vi "Activate Menu.vi"(8 "error in (no error)":errorcluster, 9 "Run mode?":bool, 10 "MenuRef":refnum<k9>, 11 "2D Plotmatrix.lvclass in":refnum<class "XY Plot Matrix.lvclass">) -> (0 "error out":errorcluster, 3 "2D Plotmatrix.lvclass out":refnum<class "XY Plot Matrix.lvclass">)   [LabVIEW 2020, in "XY Plot Matrix.lvclass"]
uses:
  <vilib>/Math Plots/2D Math Plots/XY Plot Matrix/XY Plot Matrix/XY Plot Matrix.lvclass
  e:/builds/penguin/labview/branches/2020/dev/dist/vi.lib/Math Plots/2D Math Plots/2D Plot/2D Plot/2D Plot.lvclass
  <vilib>/Math Plots/2D Math Plots/2D Plot/2D Plot/2D Plot.lvclass
panel:
  in  "Run-time Menu":T1(array[cluster])=[{"menu tag"="", "items to delete"=["APP_SC_AUTOSCALE_X", "APP_SC_AUTOSCALE_Y", "APP_SC_SMOOTH_UPDATES", "APP_SC_OPTIONAL_PLANE", "APP_SC_EXPORT", "APP_SC_SHOW_DIAGRAM", "APP_SC_EXPORT_SIMPLIFIED_IMAGE"], "new menu"=[{"item names"="Autoscale X", "item tags"="USER_SC_AUTOSCALE_X", "after item"="APP_SC_AUTOSCALE_X"}, {"item names"="Autoscale Y", "item tags"="USER_SC_AUTOSCALE_Y", "after item"="USER_SC_AUTOSCALE_X"}, {"item names"="Export Simplified Image...", "item tags"="USER_SC_EXPORT_SIMPLIFIED_IMAGE", "after item"="APP_SC_VISIBLE_ITEMS"}], "root?"=TRUE}, {"menu tag"="APP_SC_VISIBLE_ITEMS", "items to delete"=["APP_SC_PLOT_LEGEND", "APP_SC_SCALE_LEGEND", "APP_SC_GRAPH_PALETTE", "APP_SC_CURSOR_LEGEND", "APP_SC_X_SCROLLBAR", "APP_SC_X_SCALE", "APP_SC_Y_SCALE", "APP_SC_UNIT_LABEL"], "new menu"=[{"item names"="Plot Legend", "item tags"="USER_SC_PLOT_LEGEND", "after item"="APP_SC_SEPERATOR"}, {"item names"="Graph Palette", "item tags"="USER_SC_GRAPH_PALETTE", "after item"="USER_SC_SCALE_LEGEND"}], "root?"=FALSE}]
  in  "Edit-time Menu":T1(array[cluster])=[{"menu tag"="", "items to delete"=["APP_SC_AUTOSCALE_X", "APP_SC_AUTOSCALE_Y", "APP_SC_SMOOTH_UPDATES", "APP_SC_OPTIONAL_PLANE", "APP_SC_EXPORT", "APP_SC_PROPERTIES", "APP_SC_EXPORT_SIMPLIFIED_IMAGE"], "new menu"=[{"item names"="Autoscale X", "item tags"="USER_SC_AUTOSCALE_X", "after item"="APP_SC_AUTOSCALE_X"}, {"item names"="Autoscale Y", "item tags"="USER_SC_AUTOSCALE_Y", "after item"="USER_SC_AUTOSCALE_X"}, {"item names"="Export Simplified Image...", "item tags"="USER_SC_EXPORT_SIMPLIFIED_IMAGE", "after item"="APP_SC_OPTIONAL_PLANE"}, {"item names"="Properties", "item tags"="USER_SC_PROPERTIES", "after item"="APP_SC_PROPERTIES"}, {"item names"="", "item tags"="", "after item"=""}, {"item names"="", "item tags"="", "after item"=""}, {"item names"="", "item tags"="", "after item"=""}, {"item names"="", "item tags"="", "after item"=""}, {"item names"="", "item tags"="", "after item"=""}, {"item names"="Autoscale X", "item tags"="USER_SC_AUTOSCALE_X", "after item"="APP_SC_AUTOSCALE_X"}], "root?"=TRUE}, {"menu tag"="APP_SC_VISIBLE_ITEMS", "items to delete"=["APP_SC_PLOT_LEGEND", "APP_SC_SCALE_LEGEND", "APP_SC_GRAPH_PALETTE", "APP_SC_CURSOR_LEGEND", "APP_SC_X_SCROLLBAR", "APP_SC_X_SCALE", "APP_SC_Y_SCALE", "APP_SC_UNIT_LABEL"], "new menu"=[{"item names"="Plot Legend", "item tags"="USER_SC_PLOT_LEGEND", "after item"="APP_SC_SEPERATOR"}, {"item names"="Graph Palette", "item tags"="USER_SC_GRAPH_PALETTE", "after item"="USER_SC_SCALE_LEGEND"}], "root?"=FALSE}, {"menu tag"="APP_SC_ADVANCED", "items to delete"=["APP_SC_SHOW_DIAGRAM"], "new menu"=[], "root?"=FALSE}]
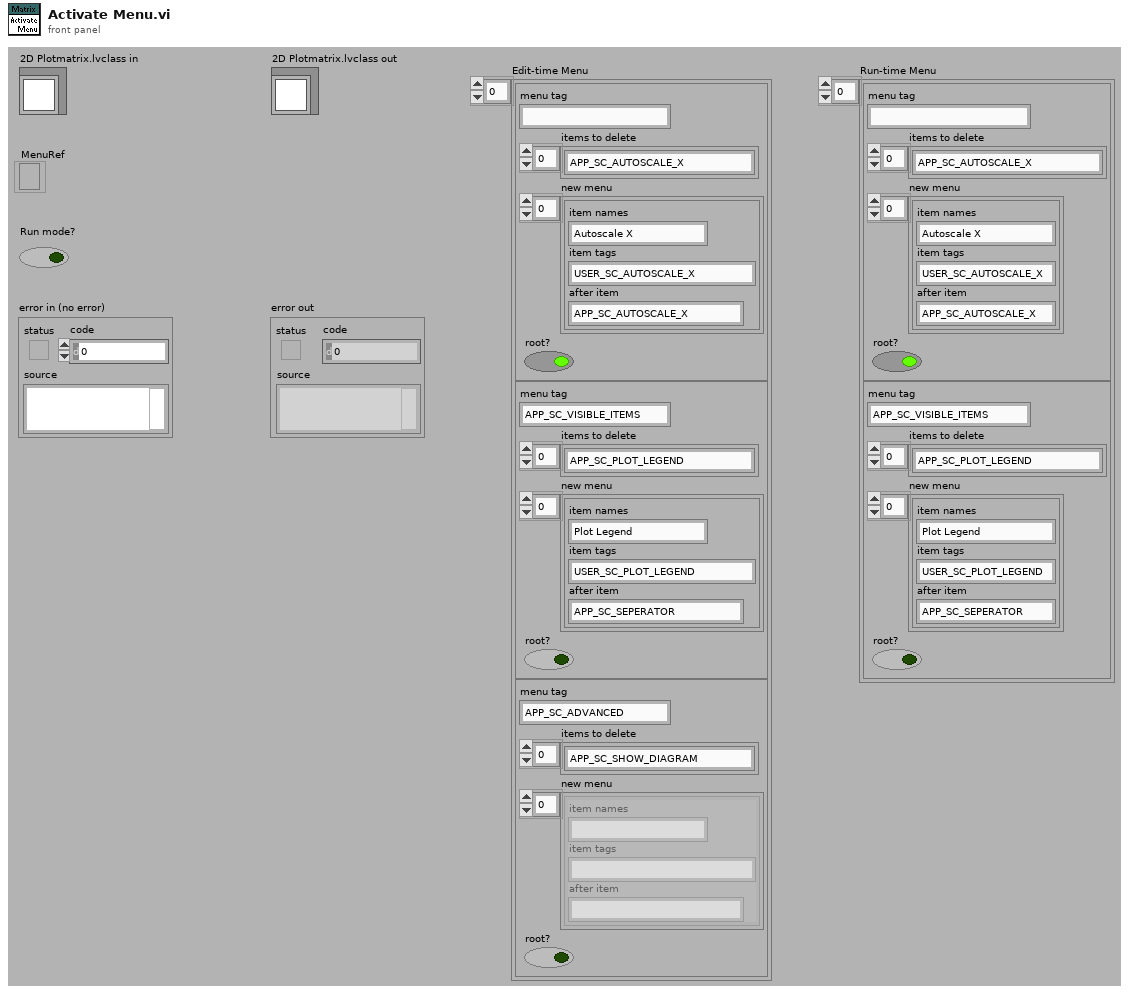
[diagram p1: front panel]
types:
  T1 = cluster{"menu tag":string, "items to delete":string[], "new menu":cluster{"item names":string, "item tags":string, "after item":string}[], "root?":bool}[]
  T2 = typedef "2D Plot.lvclass/Property Cluster.ctl" = cluster{"Graph General":T3, "Format Property":string[], "Scale Array":T4, "Cursor Property":T7, "Annotation List":T9, "Active Cursor":i32, "Active Plot":i32}
  T3 = typedef "2D Plot.lvclass/Graph General Property.ctl" = cluster{"Palette Visible":cluster{"Graph Legend":bool, "Plot Legend":bool, "Auto size":bool, "Number of Plots":u32, "X Scrollbar":bool, "Scale Legend":bool, "Cursor Legend":bool}, "Plot Area Color":cluster{"FG Color":u32, "BG Color":u32}, "Bounds Size":cluster{"Width":u32, "Height":u32}, "Plot Area Bounds":cluster{"Left":i16, "Top":i16, "Right":i16, "Bottom":i16}}
  T4 = typedef "2D Plot.lvclass/Scale Array.ctl" = T5[]
  T5 = typedef "2D Plot.lvclass/Scale Cluster.ctl" = cluster{"General":cluster{"Editable":bool, "Flipped":bool, "Mapping Mode":u8, "Visible":bool, "Style":u8, "Scale Fit":u8}, "Offset and Multiplier":T6, "Range":cluster{"Minimum":dbl, "Maximum":dbl, "Increment":dbl, "Minor Increment":dbl, "Start":dbl}, "Tick Color":cluster{"Major Color":u32, "Minor Color":u32}, "Gird Color":cluster{"Major Color":u32, "Minor Color":u32}, "Marker":cluster{"Visible":bool, "FG Color":u32, "BG Color":u32, "Font Name":string, "Font Size":u32, "Font Bold":bool, "Font Italic":bool, "Font Strikeout":bool, "Font Underline":bool}, "Name Label":cluster{"Visible":bool, "FG Color":u32, "BG Color":u32, "Font Name":string, "Font Size":u32, "Font Bold":bool, "Font Italic":bool, "Font Strikeout":bool, "Font Underline":bool, "Justification":enum16{"Left", "Center", "Right"}, "Text":string}}
  T6 = typedef "LVOffsetAndMultiplierTypeDef.ctl" = cluster{"Offset":dbl, "Multiplier":dbl}
  T7 = typedef "2D Plot.lvclass/Cursor Property.ctl" = cluster{"Cursor List":T8, "Cursor List Addtional":cluster{"Cursor Selection Color":u32, "Line Style":u8, "Line Width":u8, "Visible":bool}[]}
  T8 = typedef "LVCursorListTypeDef.ctl" = cluster{"Name":string, "Color":u32, "Style":u8, "Point Style":u8, "Name Visible":bool, "Allow Drag":bool, "Cursor Mode":u32, "Plot":i32, "Index":i32, "Position":cluster{"X":dbl, "Y":dbl}, "X Scale":u32, "Y Scale":u32, "Watch Plots":i32[], "Watch All Plots":bool, "Plot Area":i32, "Label Offset":cluster{"X":dbl, "Y":dbl}}[]
  T9 = typedef "LVAnnotationListTypeDef.ctl" = cluster{"Name":string, "Color":u32, "Style":u8, "Point Style":u8, "Name Visible":bool, "Allow Drag":bool, "Annotation Mode":u32, "Plot":i32, "Index":i32, "Position":cluster{"X":dbl, "Y":dbl}, "X Scale":u32, "Y Scale":u32, "Show Arrow":bool, "Lock Name":bool, "Plot Area":i32, "Label Offset":cluster{"X":dbl, "Y":dbl}}[]
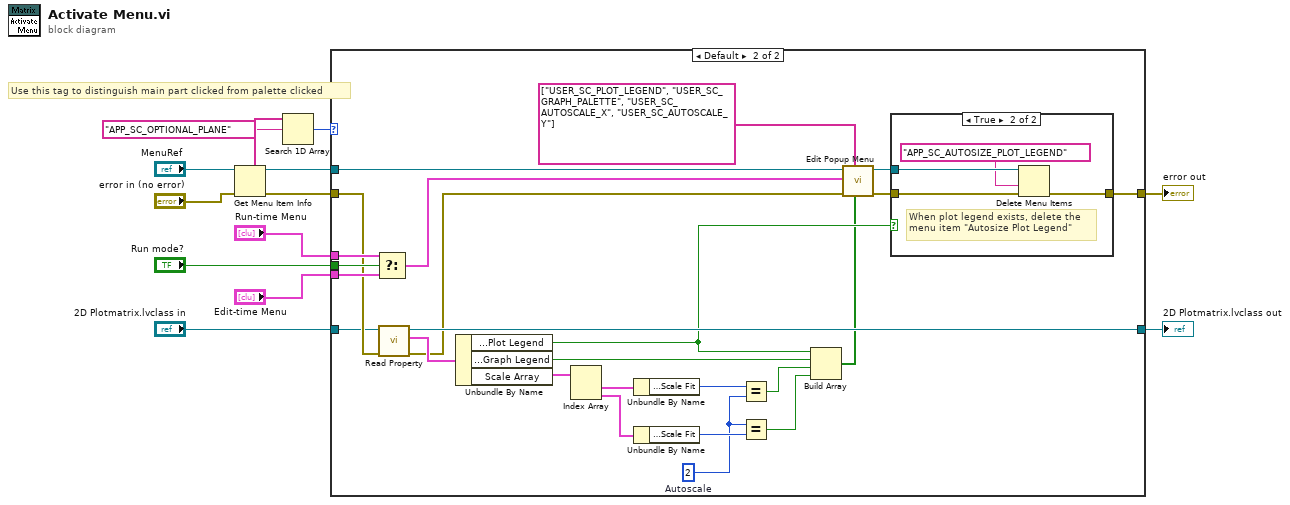
[diagram p0: block diagram]
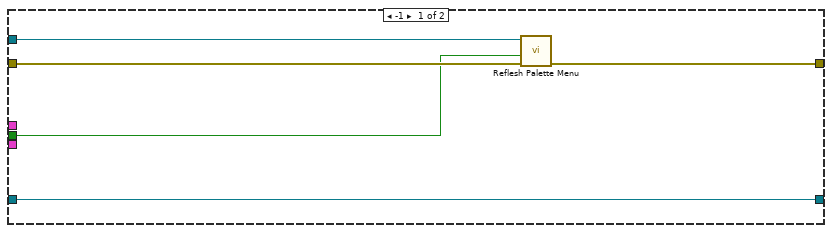
[diagram p2: hidden frame]
diagram:
  # "Use this tag to distinguish main part clicked from palette clicked"
  n1 = Get Menu Item Info(8:"error in (no error)", 11:"MenuRef") -> (0:w7:errorcluster, 3:w11:refnum<k9>, 5:w10:string[])  [unwired: 5 out]
  n2 = Search 1D Array(1D array=w10, element="APP_SC_OPTIONAL_PLANE") -> (index of element=w8:i32)  [unwired: 1 out]
  n3 = case shown="Default" w8 {
    tunnel: "2D Plotmatrix.lvclass in" -> [w18 w29]
    tunnel: "Run mode?" -> [w14 w43]
    tunnel: "Run-time Menu" -> [_ w42]
    tunnel: "Edit-time Menu" -> [_ w41]
    tunnel: w11 -> [w17 w24]
    tunnel: w7 -> [w16 w30]
    tunnel: [w15 w27] -> w2
    tunnel: [w18 w28] -> w1
    frame -1 {
      n4 = call <vilib>:"Reflesh Palette Menu.vi"("error in (no error)"=w16, "Run Mode?"=w14, "MenuRef"=w17) -> ("error out"=w15:errorcluster)  [unwired: 8 in]
    }
    frame Default {
      w33 = u8 2  # Autoscale
      n5 = Select(t=w42, s=w43, f=w41) -> (s? t:f=w25:T1)
      n6 = call <vilib>:"Read Property.vi"("error in (no error)"=w30, "2D Plot.lvclass in"=w29) -> ("error out"=w23:errorcluster, "XY Graph Property Cluster"=w31:T2, "2D Plot.lvclass out"=w28:refnum<class "XY Plot Matrix.lvclass">)  [unwired: 7 out]
      n7 = Unbundle By Name(w31) -> ("Graph General.Palette Visible.Plot Legend"=w26:bool, "Graph General.Palette Visible.Graph Legend"=w40:bool, "Scale Array"=w39:T4)
      n8 = Index Array(array=w39) -> (element #1=w38:T5, element #2=w37:T5)  [unwired: 2 in]
      n9 = Unbundle By Name(w38) -> ("General.Scale Fit"=w34:u8)
      n10 = Unbundle By Name(w37) -> ("General.Scale Fit"=w36:u8)
      n11 = Equal?(x=w34, y=w33) -> (x = y?=w32:bool)
      n12 = Equal?(x=w33, y=w36) -> (x = y?=w35:bool)
      n13 = Build Array(w26, w40, w32, w35) -> (w22:bool[])
      n14 = call <vilib>:"Edit Popup Menu.vi"("User Menu States"=w22, "User Menu Items"=string[] ["USER_SC_PLOT_LEGEND", "USER_SC_GRAPH_PALETTE", "USER_SC_AUTOSCALE_X", "USER_SC_AUTOSCALE_Y"] ("Array"), "error in (no error)"=w23, "Menu Operation Cluster"=w25, "Menu Ref In"=w24) -> ("error out"=w19:errorcluster, "Menu Ref Out"=w20:refnum<k9>)  [unwired: 5 out]
      n15 = case shown="True" w26 {
        tunnel: w19 -> [w44 w48]
        tunnel: w20 -> [_ w47]
        tunnel: [w44 w45] -> w27
        frame False {
        }
        frame True {
          # "When plot legend exists, delete the \nmenu item \"Autosize Plot Legend\""
          n16 = Delete Menu Items(6:w48, 7:"APP_SC_AUTOSIZE_PLOT_LEGEND", 9:w47) -> (0:w45:errorcluster)  [unwired: 2 out]
        }
      }
    }
  }
  "2D Plotmatrix.lvclass out" <- w1
  "error out" <- w2
